vi "AddTestSuite_TotalCountIncreases.vi"() -> ()   [LabVIEW 2019, in "TestSuiteTest.lvlib"]
uses:
  TestSuiteTest.lvlib
  c17e949e-16e6-45e4-a540-baa9e26e5c63.vi
  Constraint/IsEqual/IsEqual.lvclass
  TestSuite/TestSuite.lvclass
  Support/Support.lvlib
panel:
  out "error out":errorcluster
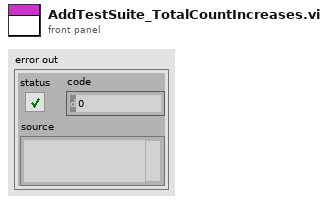
[diagram p1: front panel]
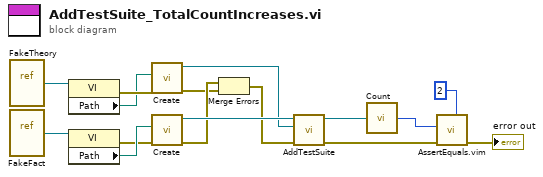
[diagram p0: block diagram]
diagram:
  n1 = vi-ref "FakeTheory.vi"() -> (w8:refnum<vi>)
  n2 = vi-ref "FakeFact.vi"() -> (w13:refnum<vi>)
  n3 = property class="VI"(reference=w8) -> (error out=w7:errorcluster, "Path"=w6:path)  [unwired: 1 in, 1 out]
  n4 = property class="VI"(reference=w13) -> (error out=w11:errorcluster, "Path"=w12:path)  [unwired: 1 in, 1 out]
  n5 = call "Create.vi"("error in (no error)"=w7, "Path"=w6) -> ("error out"=w9:errorcluster, "TestSuite"=w5:refnum<class "TestSuite.lvclass">)  [unwired: 8 in]
  n6 = call "Create.vi"("error in (no error)"=w11, "Path"=w12) -> ("error out"=w15:errorcluster, "TestSuite"=w16:refnum<class "TestSuite.lvclass">)  [unwired: 8 in]
  n7 = Merge Errors(w15, w9) -> (w10:errorcluster)
  n8 = call "AddTestSuite.vi"("error in (no error)"=w10, "TestSuite"=w5, "TestSuite in"=w16) -> ("error out"=w4:errorcluster, "TestSuite out"=w14:refnum<class "TestSuite.lvclass">)  [unwired: 7 in]
  n9 = call "Count.vi"("TestSuite In"=w14) -> ("Count"=w2:i32)
  n10 = call "AssertEquals.vim"("Expected"=2 ("Count"), "error in (no error)"=w4, "Actual"=w2) -> ("error out"=→"error out":errorcluster)  [unwired: 8 in]
